vi "Create properties (SubVI).vi"(2 "error in (no error)":errorcluster, 3 "ReplyTo":string, 4 "CorrelationId":string, 5 "ContentEncoding":string="application/json") -> (0 "error out":errorcluster, 1 "reference out":refnum<k24>)   [LabVIEW 2016]
doc: "Create properties of the message to send, following dripline protocol"
uses:
  C:/Program Files (x86)/National Instruments/LabVIEW 2016/vi.lib/Distrio/LabbitMQ/RabbitMQ.Client.dll
  Program Files (x86)/National Instruments/LabVIEW 2016/vi.lib/Distrio/LabbitMQ/RabbitMQ.Client.dll
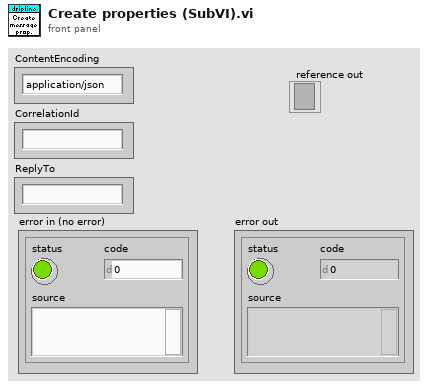
[diagram p1: front panel]
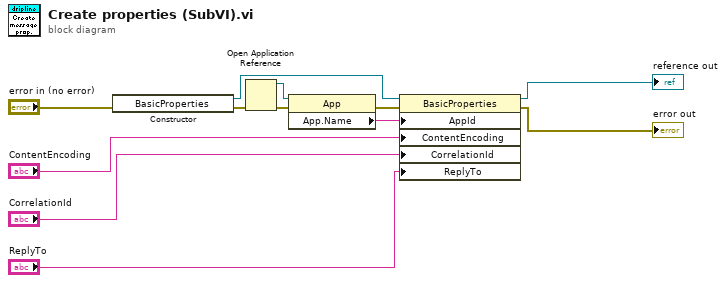
[diagram p0: block diagram]
diagram:
  n1 = constructor class="BasicProperties"(error in="error in (no error)") -> (reference out=w11:refnum<k24>, error out=w5:errorcluster)  [unwired: 2 in, 1 out]
  n2 = Open Application Reference(8:w5) -> (0:w4:errorcluster, 3:w12:refnum<vi>)  [unwired: 3 in]
  n3 = property class="App"(reference=w12, error in=w4) -> (error out=w3:errorcluster, "App.Name"=w10:string)  [unwired: 1 out]
  n4 = property class="BasicProperties"(reference=w11, error in=w3, "AppId"=w10, "ContentEncoding"="ContentEncoding", "CorrelationId"="CorrelationId", "ReplyTo"="ReplyTo") -> (reference out=→"reference out":refnum<k24>, error out=→"error out":errorcluster)
